vi "sub_stop_fgv.vi"(7 "cmd":enum16{"ini", "check", "stop"}(ring)) -> (2 "status":bool)   [LabVIEW 2018]
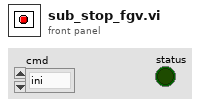
[diagram p1: front panel]
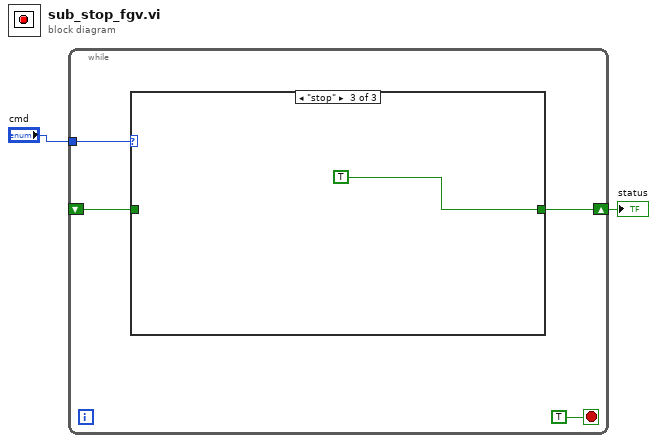
[diagram p0: block diagram]
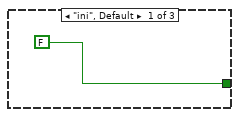
[diagram p2: hidden frame]
diagram:
  n1 = while {
    tunnel: "cmd" -> [w5]
    shift-right: [w4] -> w1
    shift-left: _ -> [w3]
    stop <- TRUE stop-if-true
    n2 = case shown="\"stop\"" w5 {
      tunnel: [FALSE w8 TRUE] -> w4
      tunnel: w3 -> [_ w8 _]
      frame "ini", Default {
      }
      frame "check" {
      }
      frame "stop" {
      }
    }
  }
  "status" <- w1
